vi "AddLabel.vi"(0 "Engine In":refnum<k7>, 5 "SequenceFile In":refnum<k7>, 7 "StepProperties":T1={"StepTypeName"="", "StepName"="", "Description"="", "Comment"="", "sequenceNameParam"="MainSequence", "Step Group"=0, "Step Index"=0, "Expression"=""} {"Step Group" items=["StepGroup_Setup", "StepGroup_Main", "StepGroup_Cleanup"]}, 11 "Error In":errorcluster) -> (4 "Engine Out":refnum<k7>, 6 "SequenceFile Out":refnum<k7>, 15 "Error Out":errorcluster)   [LabVIEW 2021, in "Create Sequence.lvlib"]
doc: "The VI inserts a label step into the sequence parameter provided and adds the description."
uses:
  Create Sequence.lvlib
  TypeDef/StepProperties.ctl
  <vilib>/addons/TestStand/_TSUtility.llb/TestStand API String Constants.ctl
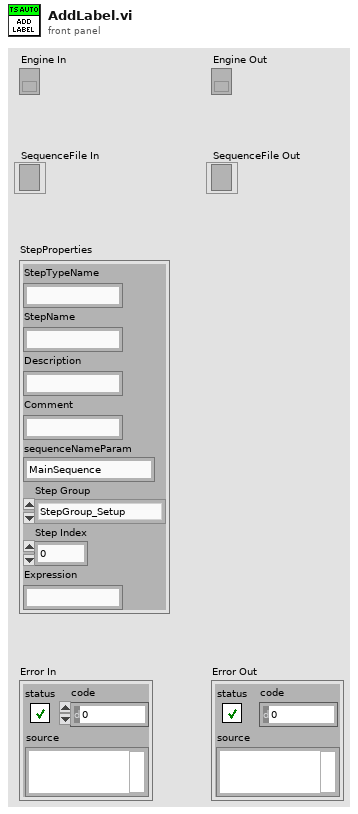
[diagram p1: front panel]
types:
  T1 = typedef "Create Sequence.lvlib/StepProperties.ctl" = cluster{"StepTypeName":string, "StepName":string, "Description":string, "Comment":string, "sequenceNameParam":string, "Step Group":i32, "Step Index":i32, "Expression":string}
  T2 = typedef "TestStand API String Constants.ctl" = enum16{"AutomationAdapterKeyName", "CVIStep_FunctionNameProp", "CVIStep_FunctionPrototypeProp", "CVIStep_ModulePathProp", "CVIStep_ModulePrjPathProp", "CVIStep_ModuleSrcPathProp", "CVIStep_ModuleTypeProp", "CVIStep_ParamsStringProp", "CVIStep_SeqContextPassProp", "DefModCback_DatabaseOptions", "DefModCback_GetReportFilePath", "DefModCback_LogToDatabase", "DefModCback_ModelOptions", "DefModCback_ModelPluginConfiguration", "DefModCback_ModelPluginOptions", "DefModCback_ModifyReportEntry", "DefModCback_ModifyReportFooter", "DefModCback_ModifyReportHeader", "DefModCback_ModifyRptEntry", "DefModCback_PostMainSequence", "DefModCback_PostUUT", "DefModCback_PostUUTLoop", "DefModCback_PreMainSequence", "DefModCback_PreUUT", "DefModCback_PreUUTLoop", "DefModCback_ProcessCleanup", "DefModCback_ProcessSetup", "DefModCback_ReportOptions", "DefModCback_TestReport", "DotNetAdapterKeyname", "ExternalCall_CallConvProp", "ExternalCall_FunctionNameProp", "ExternalCall_LibPathProp", "ExternalCall_ParametersProp", "FCParam_ArgValueProp", "FCParam_ArrayElemPassingProp", "FCParam_FlagsProp", "FCParam_NameProp", "FCParam_NumArrayElementsProp", "FCParam_NumericPassingProp", "FCParam_NumericTypeProp", "FCParam_ObjectTypeProp", "FCParam_ResultActionProp", "FCParam_StringPassingProp", "FCParam_StringSizeProp", "FCParam_TypeProp", "FeatureNamesForToggle_Enhanced_Error_Dialogs", "FeatureNamesForToggle_Python_Adapter_Debug_StepInto", "FeatureNamesForToggle_Replace_Internet_Explorer_with_CEF", "FeatureNamesForToggle_SWEEP_LOOP_ENHACEMENTS", "FeatureNamesForToggle_SupportPNGImages", "FeatureNamesForToggle_SweepLoopImprovements2021SP1", "FeatureNamesForToggle_Test_FeatureName_Incomplete", "FeatureNamesForToggle_Test_FeatureName_Prototype", "FeatureNamesForToggle_Test_FeatureName_Release", "FileContentType_AdaptersConfigFile", "FileContentType_ConfigFile", "FileContentType_CustomConfigFile", "FileContentType_GeneralEngineConfigFile", "FileContentType_ProjectFile", "FileContentType_PropertyObjectFile", "FileContentType_SearchDirectoriesConfigFile", "FileContentType_SequenceFile", "FileContentType_StationGlobalsFile", "FileContentType_TypePaletteFile", "FileContentType_TypePalettesConfigFile", "FileContentType_UsersFile", "FileContentType_WorkspaceFile", "FlexCAdapterKeyName", "FlexCStep_ExternalCallProp", "FlexCVIAdapterKeyName", "FlexLVAdapterKeyName", "FrontEndCback_LoginLogout", "GAdapterKeyName", "HTBasicAdapterKeyName", "HTBasicStep_FunctionNameProp", "HTBasicStep_ModulePathProp", "HTBasicStep_SetWorkingDirProp", "HTBasicStep_ShowAppProp", "HTBasicStep_WorkingDirPathProp", "LVAdapterKeyName", "LVStep_ModulePathProp", "LVStep_PassInBufProp", "LVStep_PassInvocInfoProp", "LVStep_PassSeqContextProp", "LVStep_ShowFrontPanelProp", "LabVIEWNXGAdapterKeyName", "Limits_HighProp", "Limits_LowProp", "Limits_NominalValueProp", "Limits_StringProp", "Limits_ThresholdTypeProp", "LoopType_Custom", "LoopType_FixedNumLoops", "LoopType_NoLoop", "LoopType_PassFailCount", "Menu_EditsSelectedFileProp", "Menu_HasEditPanelProp", "Menu_IsDimmedProp", "Menu_IsSubmenuProp", "Menu_MenuItemsProp", "Menu_NameProp", "Menu_SeparatorAboveProp", "Menu_SubstepIndexProp", "Menu_SupportsReadOnlyProp", "Menu_ToolIDProp", "NoneAdapterKeyName", "NumMeasComp_EQ", "NumMeasComp_EQTHRESHOLD", "NumMeasComp_GE", "NumMeasComp_GELE", "NumMeasComp_GELT", "NumMeasComp_GT", "NumMeasComp_GTLE", "NumMeasComp_GTLT", "NumMeasComp_LE", "NumMeasComp_LOG", "NumMeasComp_LT", "NumMeasComp_NE", "NumMeasRadix", "NumMeasThresholdType_DELTA", "NumMeasThresholdType_PERCENTAGE", "NumMeasThresholdType_PPM", "PostAction_Break", "PostAction_CallCallback", "PostAction_GotoStep", "PostAction_NextStep", "PostAction_Terminate", "Priv_Abort", "Priv_ConfigAdapter", "Priv_ConfigApp", "Priv_ConfigDatabase", "Priv_ConfigEngine", "Priv_ConfigModel", "Priv_ConfigReport", "Priv_Configure", "Priv_CtrlExecFlow", "Priv_Debug", "Priv_Develop", "Priv_EditProcessModelFiles", "Priv_EditRuntimeVariables", "Priv_EditSequenceFiles", "Priv_EditStationGlobals", "Priv_EditTemplates", "Priv_EditTypes", "Priv_EditUsers", "Priv_EditWorkspace", "Priv_Execute", "Priv_GrantAll", "Priv_LoopSelectedTests", "Priv_Operate", "Priv_RunAnySequence", "Priv_RunSelectedTests", "Priv_SaveSequenceFiles", "Priv_SinglePass", "Priv_Terminate", "Priv_UseSourceControl", "Priv_UserLoggedIn", "ProfilerMechanism_AutoSchedule", "ProfilerMechanism_Batch", "ProfilerMechanism_BatchSynchronization", "ProfilerMechanism_Lock", "ProfilerMechanism_Lot", "ProfilerMechanism_Notification", "ProfilerMechanism_Queue", "ProfilerMechanism_Rendezvous", "ProfilerMechanism_Semaphore", "ProfilerMechanism_Step", "ProfilerMechanism_StepModule", "ProfilerMechanism_StepTypeModule", "ProfilerMechanism_Suspension", "ProfilerMechanism_UUT", "ProfilerMechanism_Wait", "ProfilerOperation_Acquire", "ProfilerOperation_Break", "ProfilerOperation_Clear", "ProfilerOperation_Dequeue", "ProfilerOperation_Enqueue", "ProfilerOperation_Enter", "ProfilerOperation_Execute", "ProfilerOperation_Execution", "ProfilerOperation_Exit", "ProfilerOperation_Flush", "ProfilerOperation_Load", "ProfilerOperation_Lock", "ProfilerOperation_Pulse", "ProfilerOperation_Release", "ProfilerOperation_Rendezvous", "ProfilerOperation_Resume", "ProfilerOperation_Set", "ProfilerOperation_Test", "ProfilerOperation_Thread", "ProfilerOperation_TimeInterval", "ProfilerOperation_TimeMultiple", "ProfilerOperation_Unload", "ProfilerOperation_Unlock", "ProfilerOperation_UseResource", "ProfilerOperation_Wait", "ProfilerOutputMessageSubProperty_AdapterKeyName", "ProfilerOutputMessageSubProperty_BatchType", "ProfilerOutputMessageSubProperty_ExecutionDisplayName", "ProfilerOutputMessageSubProperty_ExecutionId", "ProfilerOutputMessageSubProperty_FileDisplayName", "ProfilerOutputMessageSubProperty_FromProcessModel", "ProfilerOutputMessageSubProperty_ModuleEnvironment", "ProfilerOutputMessageSubProperty_ModuleInputsAndOutputs", "ProfilerOutputMessageSubProperty_ModulePath", "ProfilerOutputMessageSubProperty_Name", "ProfilerOutputMessageSubProperty_NameUniquification", "ProfilerOutputMessageSubProperty_Operation", "ProfilerOutputMessageSubProperty_PackedProperties", "ProfilerOutputMessageSubProperty_ProfilerMechanism", "ProfilerOutputMessageSubProperty_ResourceAlternativeIndex", "ProfilerOutputMessageSubProperty_Sequence", "ProfilerOutputMessageSubProperty_SocketCount", "ProfilerOutputMessageSubProperty_SocketIndex", "ProfilerOutputMessageSubProperty_State", "ProfilerOutputMessageSubProperty_Step", "ProfilerOutputMessageSubProperty_StepGroup", "ProfilerOutputMessageSubProperty_StepIndex", "ProfilerOutputMessageSubProperty_ThreadDisplayName", "ProfilerOutputMessageSubProperty_ThreadId", "ProfilerOutputMessageSubProperty_TimeoutPeriod", "ProfilerOutputMessageSubProperty_UseResourceStepDescription", "PropType_CommonResults", "PropType_Error", "PropType_FCParam", "PropType_Path", "PythonAdapterKeyName", "ResultStatus_Done", "ResultStatus_Error", "ResultStatus_Failed", "ResultStatus_Looping", "ResultStatus_NoStatus", "ResultStatus_Passed", "ResultStatus_Running", "ResultStatus_Skipped", "ResultStatus_Terminated", "ResultStatus_Waiting", "Result_NumericProp", "Result_PassFailProp", "Result_StatusProp", "Result_StringProp", "RunMode_ForceFail", "RunMode_ForcePass", "RunMode_Normal", "RunMode_Skip", "RunState_LoopIndex", "RunState_LoopNumFailed", "RunState_LoopNumPassed", "RunState_SeqFileProp", "RunState_SeqProp", "RunState_StepProp", "SCStep_ActualArgsProp", "SCStep_ArgPrototypeProp", "SCStep_IgnoreTerminateProp", "SCStep_SeqFilePathExprProp", "SCStep_SeqFilePathProp", "SCStep_SeqNameExprProp", "SCStep_SeqNameProp", "SCStep_SpecifyByExprProp", "SCStep_TraceSettingProp", "SCStep_TraceSettingValDontChange", "SCStep_TraceSettingValOff", "SCStep_TraceSettingValOn", "SCStep_UseArgPrototypeProp", "SCStep_UseCurrentFileProp", "SeqContext_RunStateProp", "SeqFileCback_Load", "SeqFileCback_PostInteractive", "SeqFileCback_PostResultListEntry", "SeqFileCback_PostResults", "SeqFileCback_PostStep", "SeqFileCback_PostStepFailure", "SeqFileCback_PostStepRuntimeError", "SeqFileCback_PreInteractive", "SeqFileCback_PreStep", "SeqFileCback_Unload", "Seq_CleanupProp", "Seq_MainProp", "Seq_SetupProp", "SequenceAdapterKeyName", "StdCVIAdapterKeyName", "StepType_Action", "StepType_CallExecutable", "StepType_Goto", "StepType_Label", "StepType_LimitLoader", "StepType_MessagePopup", "StepType_MultiNumericMeasurement", "StepType_NumericMeasurement", "StepType_PassFailTest", "StepType_PropertyLoader", "StepType_PropertyLoaderEx", "StepType_SequenceCall", "StepType_Statement", "StepType_StringMeasurement", "Step_InBufProp", "Step_LimitsProp", "Step_MeasComparisonType", "Step_ResultProp", "Step_TSInfoProp", "StrMeasComp_CaseSensitive", "StrMeasComp_IgnoreCase", "TSInfo_StepAdditions", "UpdateEnumeratorsElementProperty_EnumeratorValue", "UpdateEnumeratorsElementProperty_Name", "UpdateEnumeratorsElementProperty_OldName", "VersionConstant_Company", "VersionConstant_Copyright", "VersionConstant_DisplayVersion", "VersionConstant_FullVersion", "VersionConstant_Product", "VersionConstant_Trademark", "VersionConstant_Version", "VersionConstant_YearBasedVersion"}
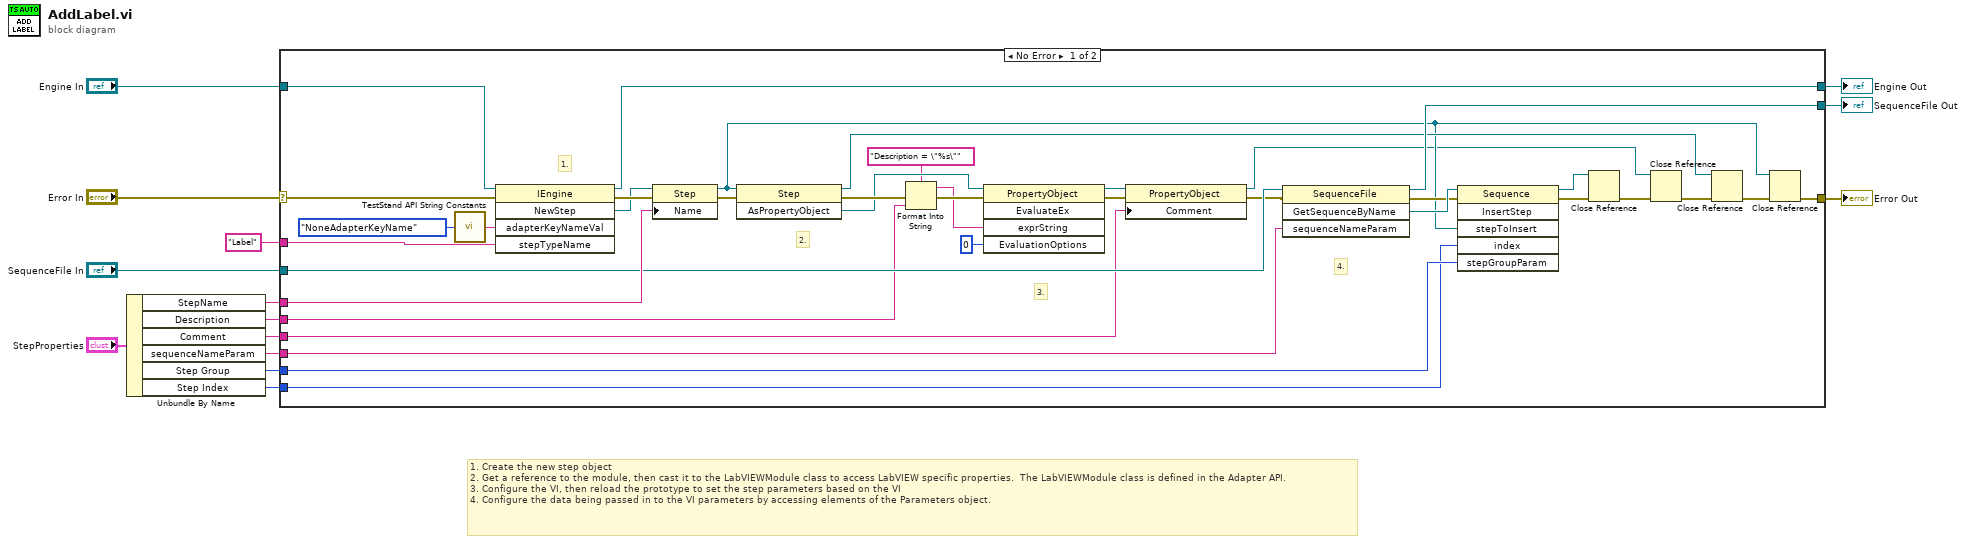
[diagram p0: block diagram]
diagram:
  # "1. Create the new step object\n2. Get a reference to the module, then cast it to the LabVIEWModule class to access LabVIEW specific properties.  The LabVIEWModule class is defined in the Adapter API.\n3. Configure the VI, then reload the prototype to set the step parameters based on the VI\n4. Configure the data being passed in to the VI parameters by accessing elements of the Parameters object."
  n1 = Unbundle By Name("StepProperties") -> ("StepName"=w6:string, "Description"=w5:string, "Comment"=w4:string, "sequenceNameParam"=w3:string, "Step Group"=w2:i32, "Step Index"=w1:i32)
  n2 = case shown="No Error" "Error In" {
    selector: "Error In" -> [w46 w54]
    tunnel: "Engine In" -> [w51 w53]
    tunnel: [w50 w53] -> w13
    tunnel: "Label" ("Step Type Name") -> [w49 _]
    tunnel: w6 -> [w48 _]
    tunnel: [w40 w52] -> w8
    tunnel: [w36 w54] -> w10
    tunnel: "SequenceFile In" -> [w41 w52]
    tunnel: w5 -> [w28 _]
    tunnel: w4 -> [w22 _]
    tunnel: w3 -> [w21 _]
    tunnel: w2 -> [w20 _]
    tunnel: w1 -> [w19 _]
    frame No Error {
      # "4."
      # "3."
      # "2."
      # "1."
      n3 = call <vilib>:"TestStand API String Constants.vi"("Constant"=TestStand_API_String_Constants."NoneAdapterKeyName" ("Adapter Type")) -> ("Value"=w32:string)  [unwired: 4 in]
      n4 = invoke class="IEngine" method="NewStep"(reference=w51, error in=w46, "adapterKeyNameVal"=w32, "stepTypeName"=w49) -> (reference out=w50:refnum<k7>, error out=w47:errorcluster, "NewStep"=w35:refnum<k7>)  [unwired: 1 in, 2 out]
      n5 = property class="Step"(reference=w35, error in=w47, "Name"=w48) -> (reference out=w30:refnum<k7>, error out=w34:errorcluster)
      n6 = invoke class="Step" method="AsPropertyObject"(reference=w30, error in=w34) -> (reference out=w33:refnum<k7>, error out=w29:errorcluster, "AsPropertyObject"=w24:refnum<k7>)  [unwired: 1 in]
      n7 = Format Into String(format string="Description = \"%s\"" ("DescriptionExpr"), error in=w29, w28) -> (resulting string=w15:string, error out=w17:errorcluster)  [unwired: 1 in]
      n8 = invoke class="PropertyObject" method="EvaluateEx"(reference=w24, error in=w17, "exprString"=w15, "EvaluationOptions"=0) -> (reference out=w23:refnum<k7>, error out=w25:errorcluster)  [unwired: 1 in, 3 out]
      n9 = property class="PropertyObject"(reference=w23, error in=w25, "Comment"=w22) -> (reference out=w26:refnum<k7>, error out=w27:errorcluster)
      n10 = invoke class="SequenceFile" method="GetSequenceByName"(reference=w41, error in=w27, "sequenceNameParam"=w21) -> (reference out=w40:refnum<k7>, error out=w42:errorcluster, "GetSequenceByName"=w43:refnum<k7>)  [unwired: 1 in, 1 out]
      n11 = invoke class="Sequence" method="InsertStep"(reference=w43, error in=w42, "stepToInsert"=w30, "index"=w19, "stepGroupParam"=w20) -> (reference out=w44:refnum<k7>, error out=w45:errorcluster)  [unwired: 1 in, 4 out]
      n12 = Close Reference(reference=w44, error in (no error)=w45) -> (error out=w38:errorcluster)
      n13 = Close Reference(reference=w26, error in (no error)=w38) -> (error out=w31:errorcluster)
      n14 = Close Reference(reference=w33, error in (no error)=w31) -> (error out=w37:errorcluster)
      n15 = Close Reference(reference=w30, error in (no error)=w37) -> (error out=w36:errorcluster)
    }
    frame Error {
    }
  }
  "Engine Out" <- w13
  "Error Out" <- w10
  "SequenceFile Out" <- w8
